vi "calc_arc_length_angle.vi"(1 "Turning Radius (in)":fxp<+/-,22,12> format="%.14g", 2 "Distance Along Arc":u16) -> (0 "arc length angle":u16)   [LabVIEW 2009]
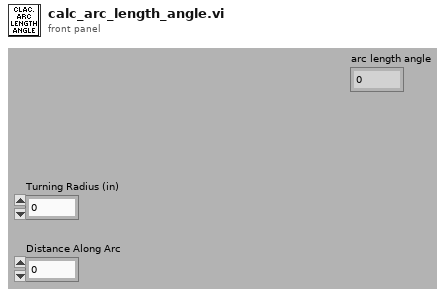
[diagram p1: front panel]
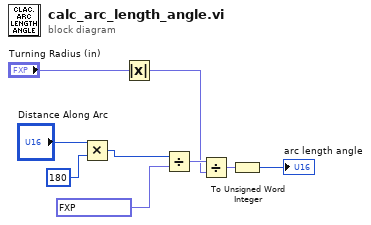
[diagram p0: block diagram]
diagram:
  n1 = Multiply(x="Distance Along Arc", y=u16 180) -> (x*y=w9:u16)
  n2 = Absolute Value(x="Turning Radius (in)") -> (abs(x)=w1:fxp<+,22,12>)
  n3 = Divide(x=w9, y=fxp<+,12,2> 3.1416015625) -> (x/y=w7:fxp<+,17,15>)
  n4 = Divide(x=w7, y=w1) -> (x/y=w3:fxp<+,16,16>)
  n5 = To Unsigned Word Integer(number=w3) -> (unsigned 16bit integer=→"arc length angle":u16)
